vi "Main_RLC.vi"() -> ()   [LabVIEW 2021]
uses:
  UNI/SECONDO ANNO/LAB 2/Pasquini/Final Project/States.ctl
  <vilib>/Analysis/NI_AALPro.lvlib
  <vilib>/Analysis/NI_AALBase.lvlib
  <vilib>/DAQmx/read.llb/DAQmx Read (Analog 1D Wfm NChan NSamp).vi
  <vilib>/Analysis/baseanly.llb/Mean (DBL).vi
  <vilib>/Analysis/6fits.llb/Confidence Interval (Exp).vi
  UNI/SECONDO ANNO/LAB 2/Pasquini/Final Project/DAQmx_Channels.ctl
  UNI/SECONDO ANNO/LAB 2/Pasquini/Final Project/DAQmx_Parameters.ctl
panel:
  in  "Sottosmorzato":bool
  in  "sovra":bool caption="Sovrasmorzato"
  in  "Subtract":bool
  in  "N offest":i32
  out "Fit XY Graph":cluster{dbl[], "Best Exponential Fit":dbl[]}[](graph)
  out "Delta RC":dbl
  out "RC":dbl
  in  "Fit Channel":enum16{"V_C", "V_R", "V_S"}(ring)
  out "Data":waveform(dbl)[](graph)
  in  "DAQ parameters":T1={"Trigger level"=1.0, "Trigger slope"=10280, "Sampling rate (Hz)"=10000.0, "Number of sampes"=1000} {"Trigger slope" items=["Rising"=10280, "Falling"=10171]; "Trigger level" scale=-10.0..10.0 scale format="%#_3g"}
  in  "Channels":T2
  in  "Exit":bool
  in  "Fit":bool
  in  "Acquire":bool
  # "RC ="
  # "±"
  # "us"
  # "Subtract mean of the last"
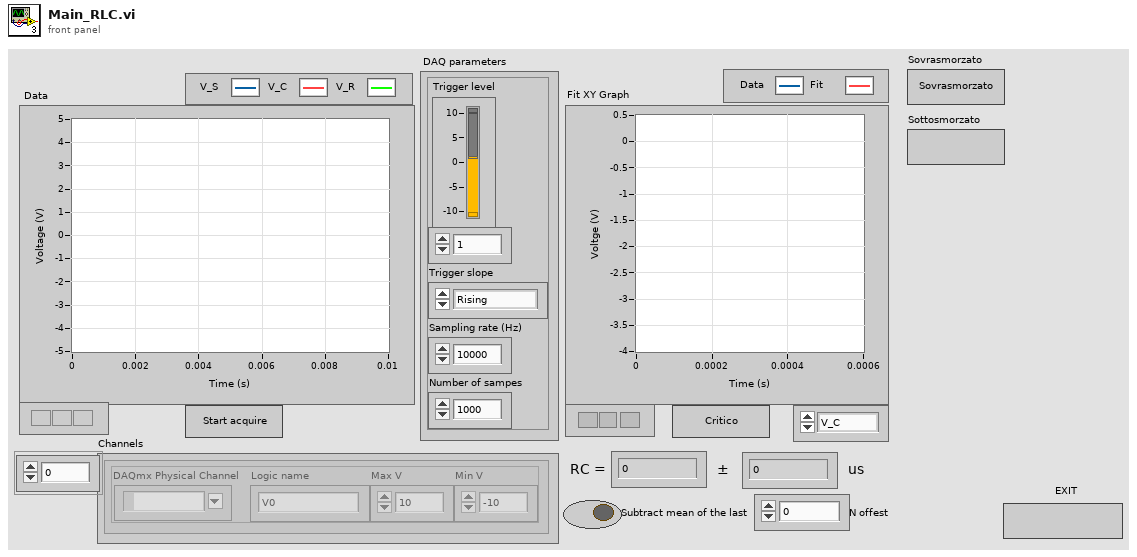
[diagram p1: front panel]
types:
  T1 = typedef "DAQmx_Parameters.ctl" = cluster{"Trigger level":dbl, "Trigger slope":u16, "Sampling rate (Hz)":dbl, "Number of sampes":i32}
  T2 = typedef "DAQmx_Channels.ctl" = cluster{"DAQmx Physical Channel":tag, "Logic name":string, "Max V":dbl, "Min V":dbl}[]
  T3 = typedef "States.ctl" = enum16{"Idle", "Acquire", "critico", "sovrasmorzato", "sottosmorzato", "Exit"}
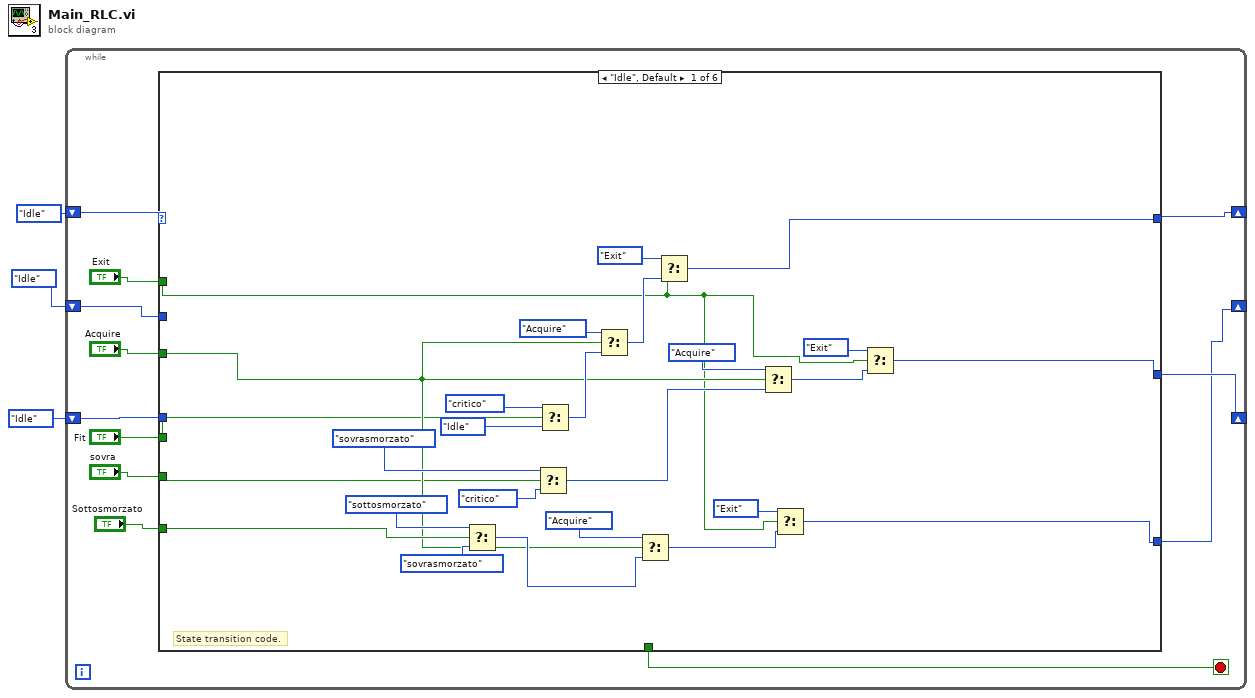
[diagram p0: block diagram]
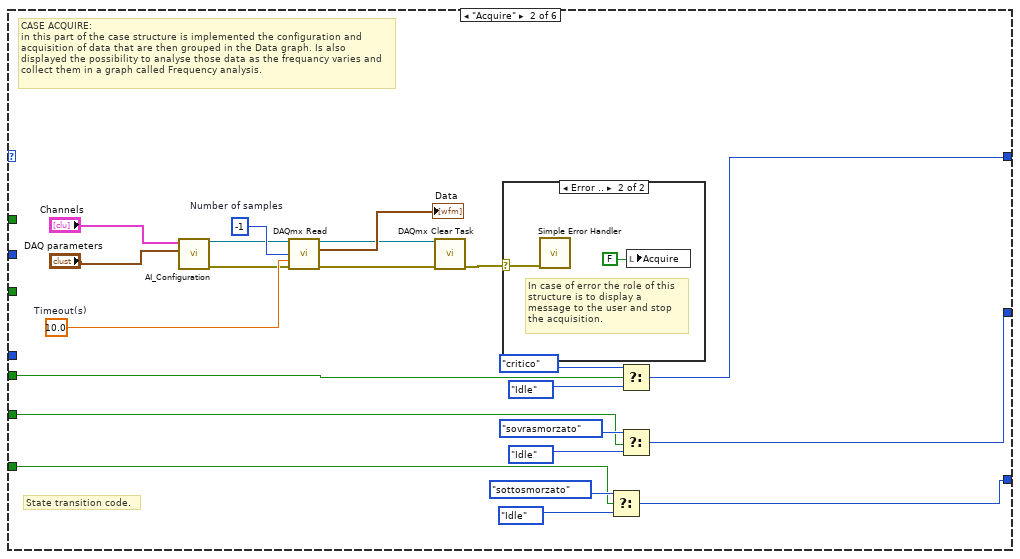
[diagram p2: hidden frame]
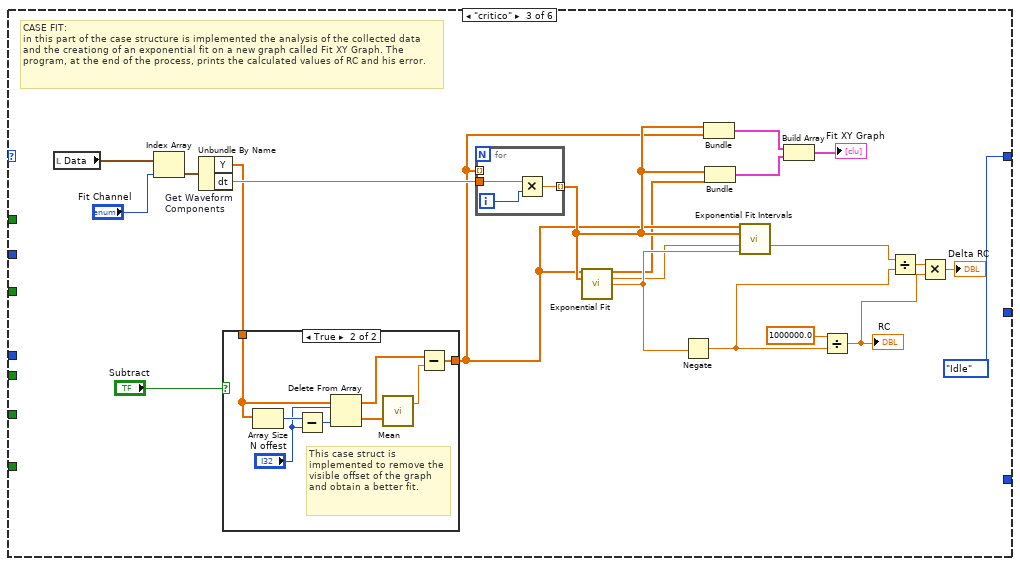
[diagram p4: hidden frame]
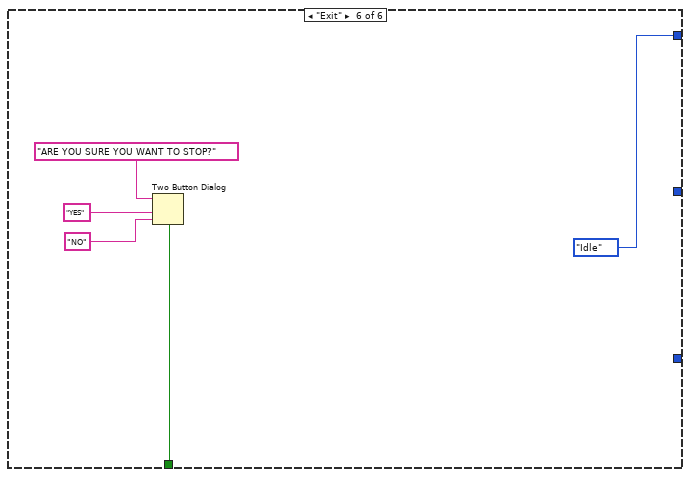
[diagram p8: hidden frame]
diagram:
  n1 = while {
    shift-right: [w11] -> _
    shift-left: States."Idle" ("States") -> [w12]
    shift-right: [w5] -> _
    shift-left: States."Idle" ("States") -> [w6]
    shift-right: [w4] -> _
    shift-left: States."Idle" ("States") -> [w7]
    stop <- w13 stop-if-true
    n2 = case shown="\"Idle\", Default" w12 {
      tunnel: "Exit" -> [w19 _ _ _ _ _]
      tunnel: "Fit" -> [w17 w63 _ _ _ _]
      tunnel: [w40 w61 States."Idle" ("states") _ _ States."Idle" ("states")] -> w11
      tunnel: [_ _ _ _ _ w102] -> w13
      tunnel: "sovra" -> [w16 w47 _ _ _ _]
      tunnel: "Sottosmorzato" -> [w34 w43 _ _ _ _]
      tunnel: "Acquire" -> [w25 _ _ _ _ _]
      tunnel: [w22 w46 _ _ _ _] -> w5
      tunnel: [w18 w42 _ _ _ _] -> w4
      tunnel: w7 -> [_ _ _ _ _ _]
      tunnel: w6 -> [_ _ _ _ _ _]
      frame "Idle", Default {
        # "State transition code."
        n3 = Select(t=States."sottosmorzato" ("states"), s=w34, f=States."sovrasmorzato" ("states")) -> (s? t:f=w26:T3)
        n4 = Select(t=States."sovrasmorzato" ("states"), s=w16, f=States."critico" ("states")) -> (s? t:f=w28:T3)
        n5 = Select(t=States."critico" ("states"), s=w17, f=States."Idle" ("states")) -> (s? t:f=w32:T3)
        n6 = Select(t=States."Acquire" ("states"), s=w25, f=w32) -> (s? t:f=w41:T3)
        n7 = Select(t=States."Acquire" ("states"), s=w25, f=w26) -> (s? t:f=w20:T3)
        n8 = Select(t=States."Exit" ("states"), s=w19, f=w41) -> (s? t:f=w40:T3)
        n9 = Select(t=States."Acquire" ("states"), s=w25, f=w28) -> (s? t:f=w23:T3)
        n10 = Select(t=States."Exit" ("states"), s=w19, f=w20) -> (s? t:f=w18:T3)
        n11 = Select(t=States."Exit" ("states"), s=w19, f=w23) -> (s? t:f=w22:T3)
      }
      frame "Acquire" {
        w58 = 10.0  # Timeout(s)
        w60 = -1  # Number of samples
        # "CASE ACQUIRE:\nin this part of the case structure is implemented the configuration and acquisition of data that are then grouped in the Data graph. Is also displayed the possibility to analyse those data as the frequancy varies and collect them in a graph called Frequency analysis."
        # "State transition code."
        n12 = call "AI_Configuration.vi"("DAQ parameters"="DAQ parameters", "Channels"="Channels") -> ("Error out"=w52:errorcluster, "Task out"=w53:refnum<k21>)  [unwired: 8 in]
        n13 = call-poly <vilib>:"DAQmx Read.vi"("task/channels in"=w53, "number of samples per channel"=w60, "timeout"=w58, "error in"=w52) -> ("task out"=w50:refnum<k21>, "data"=→"Data":waveform(dbl)[], "error out"=w59:errorcluster)  [unwired: 9 in]
        n14 = call <vilib>:"DAQmx Clear Task.vi"("task in"=w50, "error in"=w59) -> ("error out"=w57:errorcluster)  [unwired: 13 in]
        n15 = case shown="Error .." w57 {
          selector: w57 -> [_ w65]
          frame No Error {
          }
          frame Error {
            # "In case of error the role of this structure is to display a message to the user and stop the acquisition."
            n16 = call <vilib>:"Simple Error Handler.vi"("error in (no error)"=w65) -> ()  [unwired: 4 in, 5 out]
            n17 = local write "Acquire"(FALSE) -> ()
          }
        }
        n18 = Select(t=States."sottosmorzato" ("states"), s=w43, f=States."Idle" ("states")) -> (s? t:f=w42:T3)
        n19 = Select(t=States."critico" ("states"), s=w63, f=States."Idle" ("states")) -> (s? t:f=w61:T3)
        n20 = Select(t=States."sovrasmorzato" ("states"), s=w47, f=States."Idle" ("states")) -> (s? t:f=w46:T3)
      }
      frame "critico" {
        # "CASE FIT:\nin this part of the case structure is implemented the analysis of the collected data and the creationg of an exponential fit on a new graph called Fit XY Graph. The program, at the end of the process, prints the calculated values of RC and his error."
        n21 = local read "Data"() -> (w86:waveform(dbl)[])
        n22 = Index Array(array=w86, index="Fit Channel") -> (element=w84:waveform(dbl))
        n23 = Unbundle By Name "Get Waveform Components"(w84) -> ("Y"=w74:dbl[], "dt"=w83:dbl)
        n24 = case shown="True" "Subtract" {
          tunnel: w74 -> [w87 w95]
          tunnel: [w87 w88] -> w70
          frame False {
          }
          frame True {
            # "This case struct is implemented to remove the visible offset of the graph and obtain a better fit."
            n25 = Array Size(array=w95) -> (size(s)=w94:i32)
            n26 = Subtract(x=w94, y="N offest") -> (x-y=w93:i32)
            n27 = Delete From Array(array=w95, length="N offest", index=w93) -> (deleted portion=w91:dbl[], array with subset deleted=w90:dbl[])
            n28 = call-poly <vilib>:"Mean.vi"("X"=w91) -> ("mean"=w89:dbl)  [unwired: 1 out]
            n29 = Subtract(x=w90, y=w89) -> (x-y=w88:dbl[])
          }
        }
        n30 = for {
          tunnel: w83 -> [w98]
          tunnel: [w97] -> w76 mode=indexing
          tunnel: w70 -> [_] mode=indexing
          i -> [w96]
          n31 = Multiply(x=w98, y=w96) -> (x*y=w97:dbl)
        }
        n32 = call <vilib>:"Exponential Fit.vi"("Y"=w70, "X"=w76) -> ("Best Exponential Fit"=w66:dbl[], "amplitude"=w67:dbl, "damping"=w82:dbl)  [unwired: 8 in, 3 out]
        n33 = Negate(x=w82) -> (-x=w79:dbl)
        n34 = Bundle(w76, "Y"=w70) -> (w72:cluster{dbl[], "Y":dbl[]})  [unwired: 1 in]
        n35 = Bundle(w76, "Best Exponential Fit"=w66) -> (w75:cluster{dbl[], "Best Exponential Fit":dbl[]})  [unwired: 1 in]
        n36 = call-poly <vilib>:"Exponential Fit Intervals.vi"("Y"=w70, "X"=w76, "amplitude"=w67, "damping"=w82) -> ("delta damping"=w80:dbl)  [unwired: 7 in, 4 out]
        n37 = Build Array(w72, w75) -> (→"Fit XY Graph":cluster{dbl[], "Best Exponential Fit":dbl[]}[])
        n38 = Divide(x=1000000.0, y=w79) -> (x/y=w77:dbl)
        "RC" <- w77
        n39 = Divide(x=w80, y=w79) -> (x/y=w78:dbl)
        n40 = Multiply(x=w78, y=w77) -> (x*y=→"Delta RC":dbl)
      }
      frame "sovrasmorzato" {
      }
      frame "sottosmorzato" {
      }
      frame "Exit" {
        n41 = Two Button Dialog(message="ARE YOU SURE YOU WANT TO STOP?", 1:"NO" ("F button name (\"Cancel\")"), 2:"YES" ("T button name (\"OK\")")) -> (T button?=w102:bool)
      }
    }
  }
